vi "차선 0 제거.vi"(1 "추가된 배열":dbl[][](array[numeric])) -> (0 "제거된 배열":dbl[][](array[numeric]))   [LabVIEW 2016]
panel:
  out "삭제된 부분":dbl[](array[numeric])
  out "제거 갯수":i8
  out "반복횟수":i32
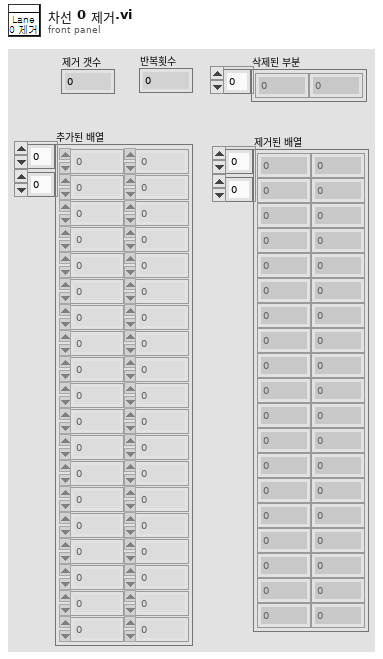
[diagram p1: front panel]
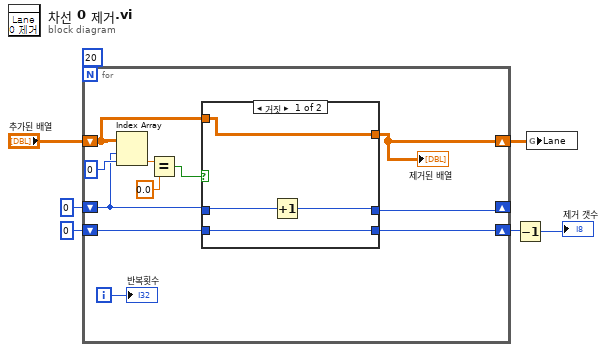
[diagram p0: block diagram]
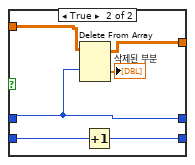
[diagram p2: hidden frame]
diagram:
  n1 = for {
    N: 20 -> [_]
    shift-right: [w16] -> w5
    shift-left: "추가된 배열" -> [w13]
    shift-right: [w14] -> w2
    shift-left: i8 0 -> [w15]
    shift-right: [w11] -> _
    shift-left: i8 0 -> [w9]
    i -> [w10]
    n2 = Index Array(array=w13, index (row)=w9, index (col)=0 ("비활성화된 인덱스 (열)")) -> (element=w18:dbl)
    n3 = Equal?(x=w18, y=0.0) -> (x = y?=w8:bool)
    n4 = case shown="거짓" w8 {
      tunnel: w13 -> [w21 w28]
      tunnel: [w21 w27] -> w16
      tunnel: w9 -> [w20 w23]
      tunnel: w15 -> [w22 w25]
      tunnel: [w22 w26] -> w14
      tunnel: [w19 w23] -> w11
      frame False {
        n5 = Increment(x=w20) -> (x+1=w19:i8)
      }
      frame True {
        n6 = Delete From Array(array=w28, index (row)=w23) -> (deleted portion=→"삭제된 부분":dbl[], array with subset deleted=w27:dbl[][])  [unwired: 2 in]
        n7 = Increment(x=w25) -> (x+1=w26:i8)
      }
    }
    "제거된 배열" <- w16
    "반복횟수" <- w10
  }
  n8 = Decrement(x=w2) -> (x-1=→"제거 갯수":i8)
  n9 = global write "[GV]_Vision Lane.vi" "Lane"(w5) -> ()
